vi "Export Configuration RTM.vi"(8 "error in (no error)":errorcluster, 11 "Node Ptr":u64 format="%.0x") -> (0 "error out":errorcluster)   [LabVIEW 2017, in "SLSC Switch System Explorer.lvlib"]
uses:
  SLSC Switch System Explorer.lvlib
  Scripting/SLSC Switch Scripting.lvlib
panel:
  in  "Tag":string
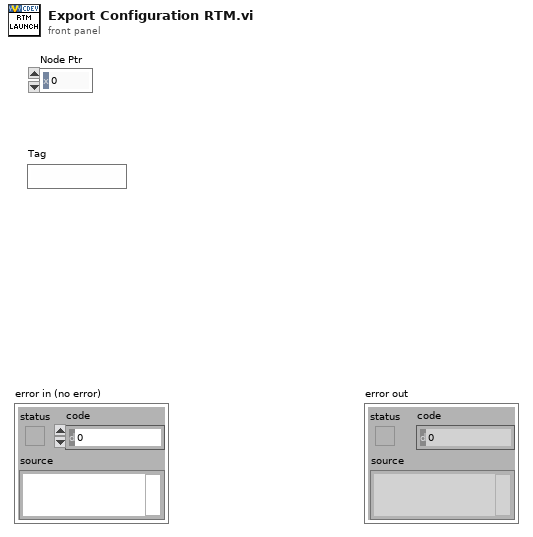
[diagram p1: front panel]
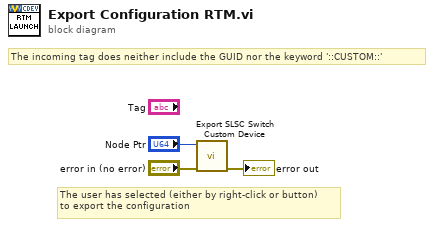
[diagram p0: block diagram]
diagram:
  # "The user has selected (either by right-click or button)\nto export the configuration"
  # "The incoming tag does neither include the GUID nor the keyword '::CUSTOM::'"
  n1 = call "Export SLSC Switch Custom Device.vi"("error in (no error)"="error in (no error)", "SLSC Switch Custom Device Ref in"="Node Ptr") -> ("error out"=→"error out":errorcluster)  [unwired: 8 in, 1 out]
